vi "Command_Shoot.vi"(0 "Startup":bool, 2 "Timeout":dbl) -> (6 "Reint":bool, 7 "Completed":bool, 10 "Output":bool)   [LabVIEW 2020]
uses:
  Auto Utilities/Command_Execution_State.ctl
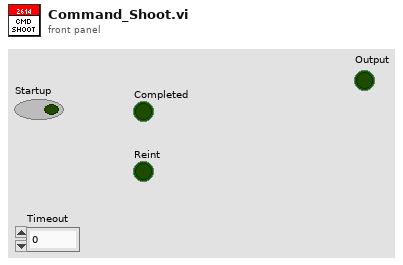
[diagram p1: front panel]
types:
  T1 = typedef "Command_Execution_State.ctl" = enum16{"Initialize", "Execute", "Finish"}
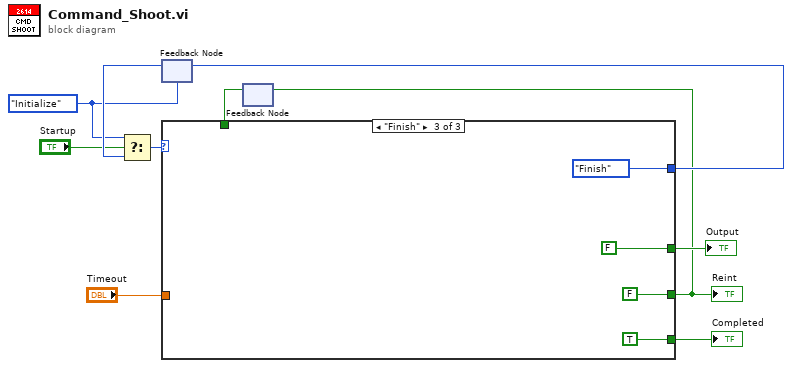
[diagram p0: block diagram]
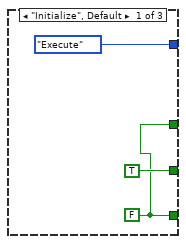
[diagram p2: hidden frame]
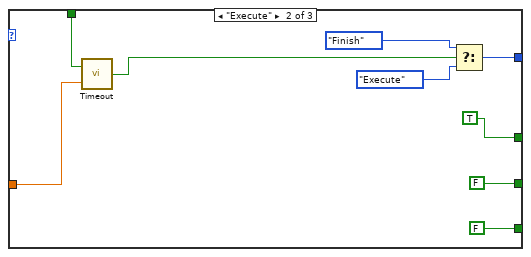
[diagram p3: hidden frame]
diagram:
  w5 = Command_Execution_State."Initialize" ("Play State")
  n1 = feedback #1(w5) -> (w8:T1)
  n2 = Select(t=w5, s="Startup", f=w8) -> (s? t:f=w10:T1)
  n3 = feedback #2() -> (w4:bool)  [unwired: 1 in]
  n4 = case shown="\"Finish\"" w10 {
    tunnel: [Command_Execution_State."Execute" ("Play State") w18 Command_Execution_State."Finish" ("Play State")] -> w9
    tunnel: [w11 FALSE TRUE] -> w7
    tunnel: [TRUE FALSE FALSE] -> w1
    tunnel: w4 -> [_ w20 _]
    tunnel: "Timeout" -> [_ w19 _]
    tunnel: [w11 TRUE FALSE] -> w2
    frame "Initialize", Default {
      w11 = FALSE
    }
    frame "Execute" {
      n5 = call "Timeout.vi"("Timeout"=w19, "Initialize"=w20) -> ("Timed Out?"=w15:bool)
      n6 = Select(t=Command_Execution_State."Finish" ("Play State"), s=w15, f=Command_Execution_State."Execute" ("Play State")) -> (s? t:f=w18:T1)
    }
    frame "Finish" {
    }
  }
  "Completed" <- w7
  "Reint" <- w1
  "Output" <- w2
  n7 = feedback-in #1(w9) -> ()
  n8 = feedback-in #2(w1) -> ()
